vi "Write Name.vi"(7 "Linked List ID":string, 8 "error in (no error)":errorcluster, 10 "Name":string, 11 "Linked List in":refnum<class "Linked List.lvclass">) -> (0 "error out":errorcluster, 3 "Linked List out":refnum<class "Linked List.lvclass">)   [LabVIEW 2017, in "Linked Lists.lvlib" / "Linked List.lvclass"]
uses:
  <vilib>/gpm_packages/@cs/linked-list/Source/Linked List/Linked List/Linked List.lvclass
  <vilib>/gpm_packages/@cs/linked-list/Source/Linked List/Linked List Definition/Linked List Definition.lvclass
  <vilib>/gpm_packages/@cs/linked-list/Source/Linked List/Linked List/Linked List.lvclass/Linked List.ctl
  <vilib>/gpm_packages/@cs/lookup-table/Source/LookupTable/LookupTable.lvclass/LookupTable.ctl
  1a4611dd-03d2-4be4-9f29-518b068c0f16.vi
  6851e142-b771-4e18-a96a-cdb514326faf.vi
  <vilib>/gpm_packages/@cs/lookup-table/Source/LookupTable/Read Table Reference.vi
  1a4611dd-03d2-4be4-9f29-518b068c0f16.vi/10631ca8-2613-4837-8efb-6d72a554eb47.vi
  6851e142-b771-4e18-a96a-cdb514326faf.vi/754c9cd5-5cd0-42b0-ae1b-07db77e0750d.vi
  <vilib>/gpm_packages/@cs/lookup-table/Source/LookupTable/LookupTable.lvclass
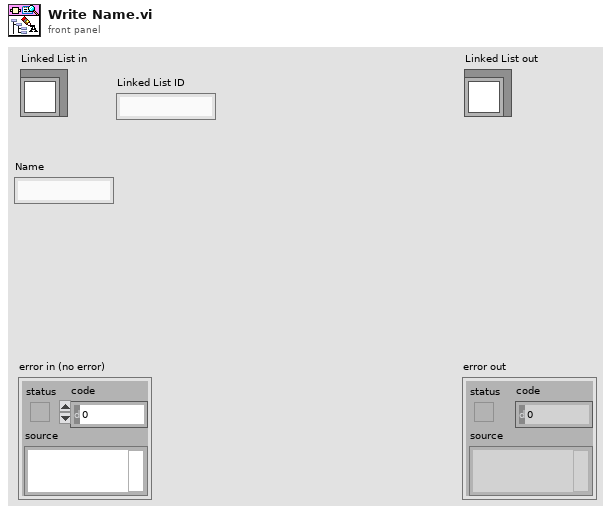
[diagram p1: front panel]
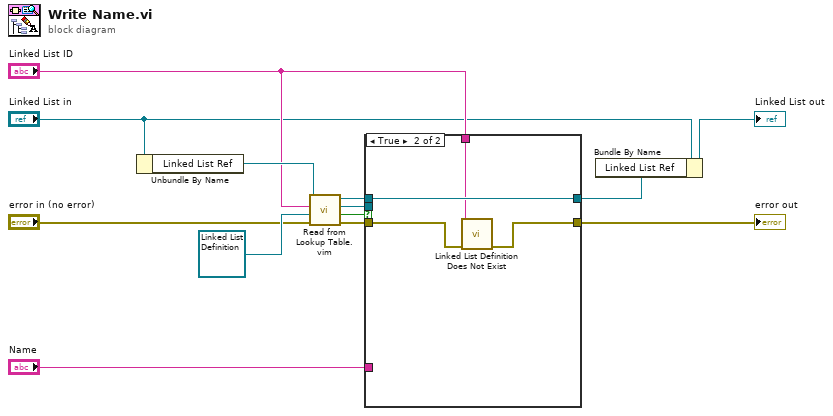
[diagram p0: block diagram]
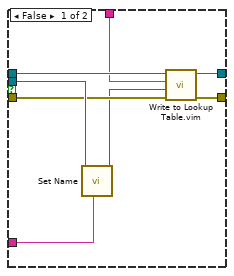
[diagram p2: hidden frame]
diagram:
  n1 = Unbundle By Name("Linked List in") -> ("Linked List Ref"=w9:refnum<data-value>)
  n2 = call "Read from Lookup Table.vim"("error in (no error)"="error in (no error)", "Type"=refnum<class "Linked List Definition.lvclass"> refnum ("Linked Lists.lvlib:Linked List Definition.lvclass"), "Item Name"="Linked List ID", "LookupTable Reference"=w9) -> ("error out"=w7:errorcluster, "Not Found?"=w1:bool, "Value"=w11:refnum<class "Linked List Definition.lvclass">, "LookupTable Reference Out"=w8:refnum<data-value>)  [unwired: 4 in]
  n3 = case shown="True" w1 {
    tunnel: w11 -> [w21 _]
    tunnel: "Name" -> [w20 _]
    tunnel: w8 -> [w19 w23]
    tunnel: w7 -> [w18 w25]
    tunnel: "Linked List ID" -> [w16 w22]
    tunnel: [w15 w23] -> w4
    tunnel: [w14 w24] -> w2
    frame False {
      n4 = call <vilib>:"Set Name.vi"("Name"=w20, "Linked List Definition in"=w21) -> ("Linked List Definition out"=w17:refnum<class "Linked List Definition.lvclass">)  [unwired: 9 in]
      n5 = call "Write to Lookup Table.vim"("error in (no error)"=w18, "Item"=w17, "Item Name"=w16, "LookupTable Reference"=w19) -> ("error out"=w14:errorcluster, "LookupTable Reference Out"=w15:refnum<data-value>)  [unwired: 5 in, 1 out]
    }
    frame True {
      n6 = call <vilib>:"Linked List Definition Does Not Exist.vi"("Error In"=w25, "Unique ID"=w22) -> ("Error Out"=w24:errorcluster)  [unwired: 9 in]
    }
  }
  "error out" <- w2
  n7 = Bundle By Name(cluster="Linked List in", "Linked List Ref"=w4) -> (→"Linked List out":refnum<class "Linked List.lvclass">)
